vi "Set VI Properties.vi"(9 "Front Panel Controls":T1, 11 "VI Data in":T2[](array[typedef])) -> (3 "VI Data out":T2[](array[typedef]))   [LabVIEW 2023, in "VI Properties Editor.lvlib"]
doc: "Sets all new VI properties of the VI identified by <B>VI Selected</B>."
uses:
  VI Properties Editor.lvlib
  CTLs/VI Data.ctl
  CTLs/VI Properties.ctl
  <vilib>/picture/picture.llb/imagedata.ctl
  CTLs/Control Properties.ctl
  CTLs/VI Properties Editor Front Panel Controls.ctl
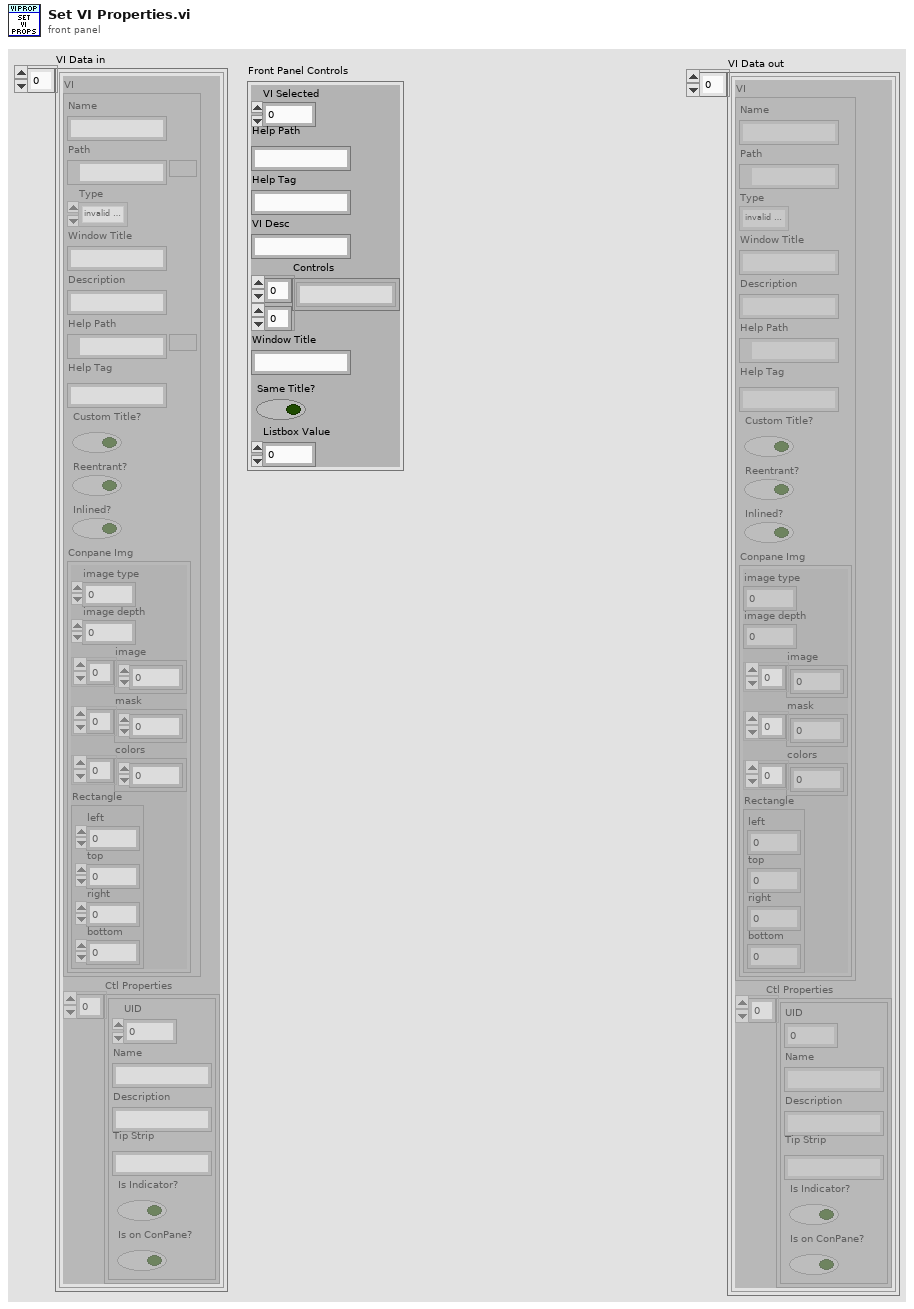
[diagram p1: front panel]
types:
  T1 = typedef "VI Properties Editor.lvlib/VI Properties Editor Front Panel Controls.ctl" = cluster{"VI Selected":i32, "Help Path":string, "Help Tag":string, "VI Desc":string, "Controls":string[][], "Window Title":string, "Same Title?":bool, "Listbox Value":i32}
  T2 = typedef "VI Properties Editor.lvlib/VI Data.ctl" = cluster{"VI":T3, "Ctl Properties":T5[]}
  T3 = typedef "VI Properties Editor.lvlib/VI Properties.ctl" = cluster{"Name":string, "Path":path, "Type":enum32{"invalid VI type", "Standard VI", "Control VI", "Global VI", "Polymorphic VI", "Configuration VI", "SubSystem", "Facade VI", "Method VI", "Statechart Diagram VI"}, "Window Title":string, "Description":string, "Help Path":path, "Help Tag":string, "Custom Title?":bool, "Reentrant?":bool, "Inlined?":bool, "Conpane Img":T4}
  T4 = typedef "imagedata.ctl" = cluster{"image type":i32, "image depth":i32, "image":u8[], "mask":u8[], "colors":u32[], "Rectangle":cluster{"left":i16, "top":i16, "right":i16, "bottom":i16}}
  T5 = typedef "VI Properties Editor.lvlib/Control Properties.ctl" = cluster{"UID":i32, "Name":string, "Description":string, "Tip Strip":string, "Is Indicator?":bool, "Is on ConPane?":bool}
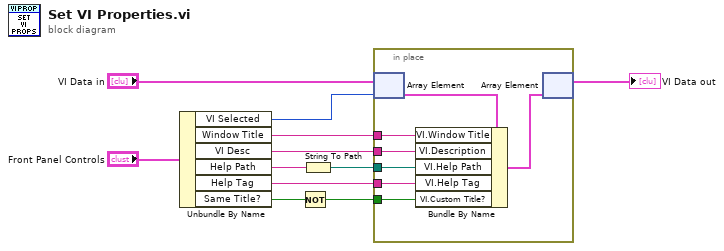
[diagram p0: block diagram]
diagram:
  n1 = Unbundle By Name("Front Panel Controls") -> ("VI Selected"=w7:i32, "Window Title"=w6:string, "VI Desc"=w5:string, "Help Path"=w4:string, "Help Tag"=w3:string, "Same Title?"=w2:bool)
  n2 = Not(x=w2) -> (.not. x?=w1:bool)
  n3 = String To Path(string=w4) -> (path=w9:path)
  n4 = in-place {
    in-place-border: w5 -> [w17]
    in-place-border: w9 -> [w16]
    in-place-border: w3 -> [w15]
    in-place-border: w6 -> [w13]
    in-place-border: w1 -> [w12]
    n5 = in-place-array #1("VI Data in", w7) -> (w18:T2)
    n6 = Bundle By Name(cluster=w18, "VI.Window Title"=w13, "VI.Description"=w17, "VI.Help Path"=w16, "VI.Help Tag"=w15, "VI.Custom Title?"=w12) -> (w14:T2)
    n7 = in-place-array #1(w14) -> (→"VI Data out":T2[])  [unwired: 1 out]
  }
